vi "Check_and_rewrite_file.vi"(0 "Filename":path, 7 "Present Channels only":bool, 9 "Present Channels":string[](array[string]), 11 "Start of read offset (chars.: 0)":i32) -> (4 "exists?":bool, 6 "Merged Channels":string[](array[string]), 8 "Start of data (bytes)":i32, 10 "No of bytes/row (approx)":i32, 14 "Current file size (bytes)":i32, 15 "Merged?":bool)   [LabVIEW 2014]
uses:
  Anemometry/Anemometry Sub Vis/Globals/Constants_global.vi
panel:
  in  "stop":bool
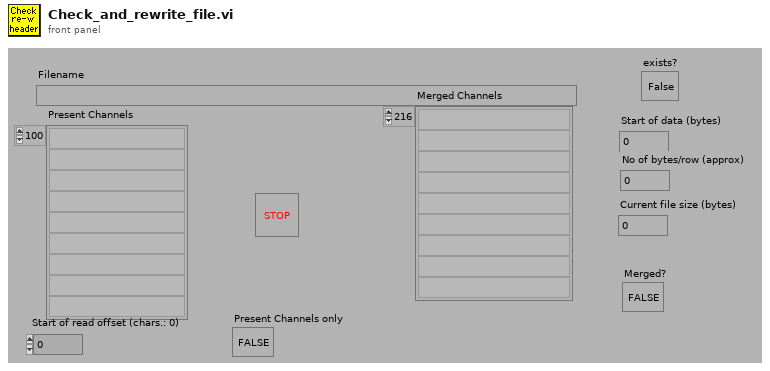
[diagram p1: front panel]
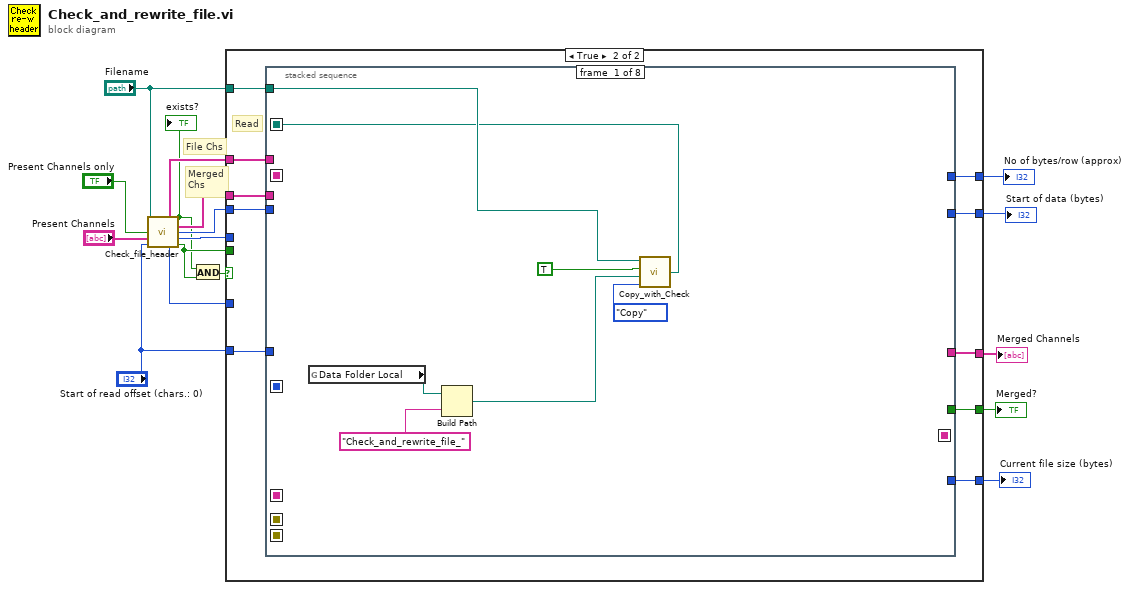
[diagram p0: block diagram]
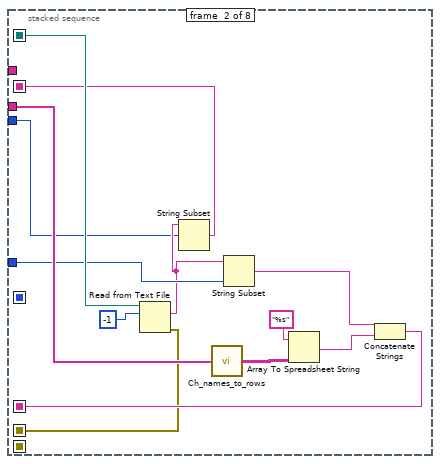
[diagram p3: hidden frame]
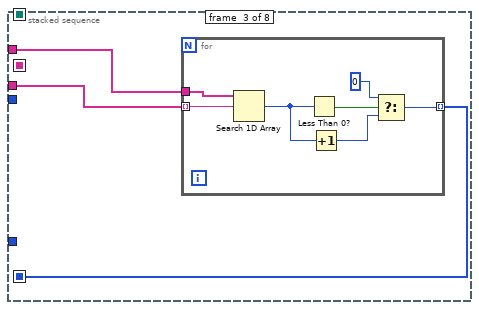
[diagram p4: hidden frame]
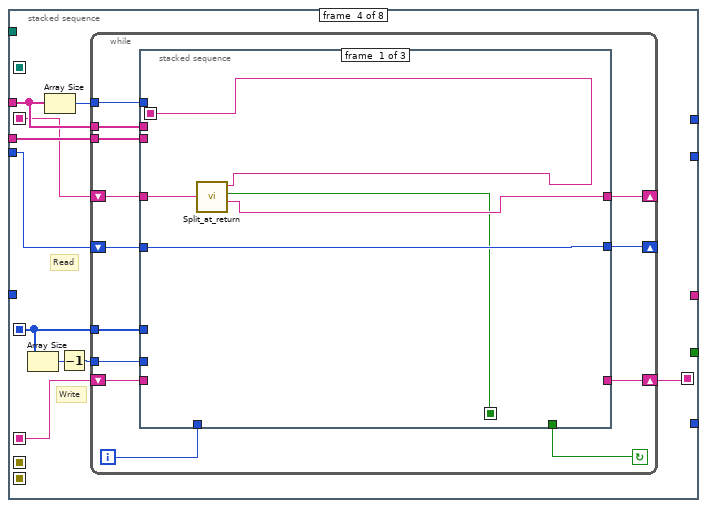
[diagram p5: hidden frame]
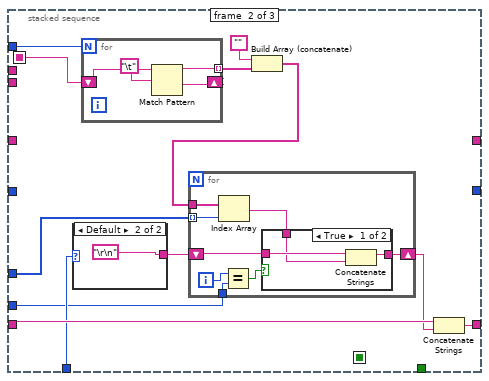
[diagram p6: hidden frame]
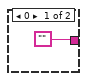
[diagram p7: hidden frame]
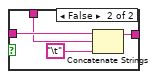
[diagram p8: hidden frame]
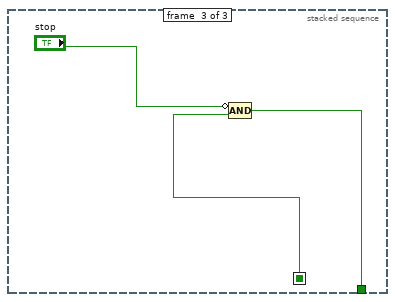
[diagram p9: hidden frame]
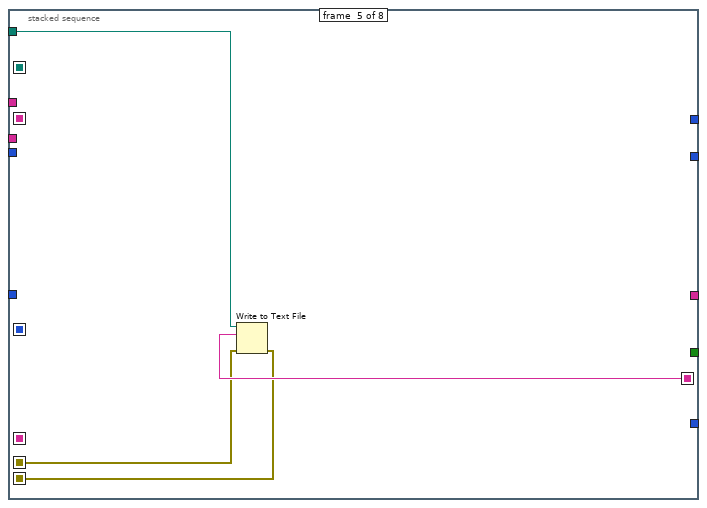
[diagram p10: hidden frame]
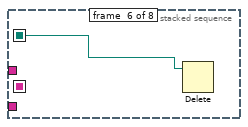
[diagram p11: hidden frame]
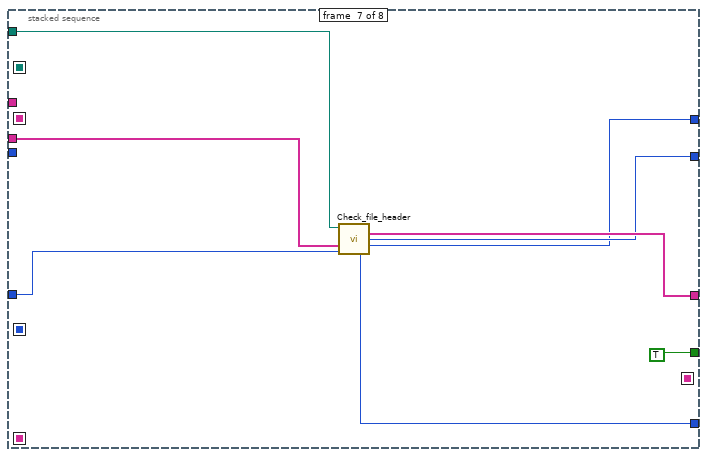
[diagram p12: hidden frame]
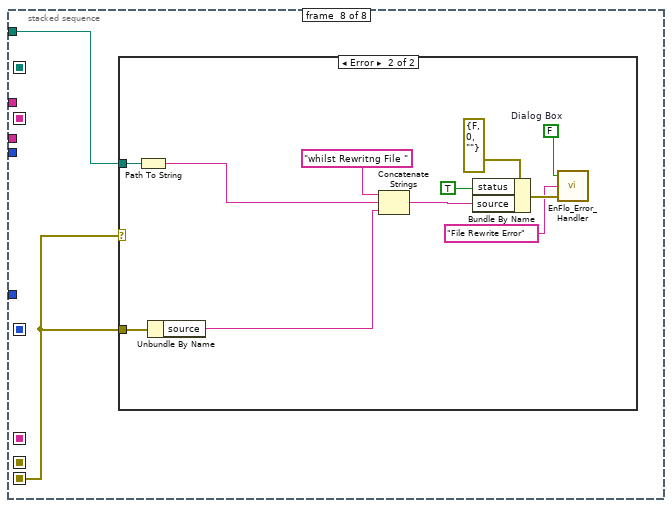
[diagram p13: hidden frame]
diagram:
  # "Merged\nChs"
  # "File Chs"
  n1 = call "Check_file_header.vi"("Filename"="Filename", "Present Channels only"="Present Channels only", "Present Channels"="Present Channels", "Start of read offset (chars.: 0)"="Start of read offset (chars.: 0)") -> ("File Channels"=w5:string[], "exists?"=w4:bool, "Merged Channels"=w11:string[], "Start of data (bytes)"=w10:i32, "No of bytes/row (approx)"=w9:i32, "Current file size (bytes)"=w8:i32, "Merged?"=w12:bool)  [unwired: 5 out]
  "exists?" <- w4
  n2 = And(x=w4, y=w12) -> (x .and. y?=w1:bool)
  n3 = case shown="True" w1 {
    tunnel: [w21 w30] -> w17
    tunnel: [w22 w29] -> w16
    tunnel: [w19 w27] -> w15
    tunnel: [w20 w28] -> w14
    tunnel: [w18 w26] -> w13
    tunnel: w12 -> [w22 _]
    tunnel: w11 -> [w21 w31]
    tunnel: w10 -> [w20 w24]
    tunnel: w9 -> [w19 _]
    tunnel: w8 -> [w18 _]
    tunnel: "Start of read offset (chars.: 0)" -> [_ w25]
    tunnel: w5 -> [_ w23]
    tunnel: "Filename" -> [_ w32]
    frame False {
    }
    frame True {
      # "Read"
      n4 = stacked-sequence {
        seq-local: [w34 _ _ _ _ _ _ _] -> [_ w48 _ _ _ w131 _ _]
        seq-local: [_ _ w53 _ _ _ _ _] -> [_ _ _ w65 _ _ _ _]
        seq-local: [_ _ _ w68 _ _ _ _] -> [_ _ _ _ w130 _ _ _]
        seq-local: [_ w47 _ _ _ _ _ _] -> [_ _ _ w66 _ _ _ _]
        seq-local: [_ w41 _ _ _ _ _ _] -> [_ _ _ w67 _ _ _ _]
        seq-local: [_ w40 _ _ _ _ _ _] -> [_ _ _ _ w128 _ _ _]
        seq-local: [_ _ _ _ w127 _ _ _] -> [_ _ _ _ _ _ _ w140]
        tunnel: w32 -> [w36 _ _ _ w129 _ w138 w141]
        tunnel: w31 -> [_ w50 w55 w69 _ _ w139 _]
        tunnel: [_ _ _ _ _ _ w137 _] -> w30
        tunnel: [_ _ _ _ _ _ TRUE _] -> w29
        tunnel: [_ _ _ _ _ _ w135 _] -> w28
        tunnel: [_ _ _ _ _ _ w134 _] -> w27
        tunnel: [_ _ _ _ _ _ w133 _] -> w26
        tunnel: w25 -> [_ w45 _ _ _ _ w132 _]
        tunnel: w24 -> [_ w42 _ w72 _ _ _ _]
        tunnel: w23 -> [_ _ w54 w70 _ _ _ _]
        frame #0 {
          n5 = global read "Constants_global.vi" "Data Folder Local"() -> (w39:path)
          n6 = Build Path(base path=w39, name or relative path="Check_and_rewrite_file_") -> (appended path=w35:path)
          n7 = call "Copy_with_Check.vi"("Mode"=enum16{"Move", "Copy"}."Copy", "Target Path"=w35, "Variable Target?"=TRUE, "Source Path"=w36) -> ("Pathname Out"=w34:path)
        }
        frame #1 {
          n8 = Read from Text File(file (use dialog)=w48, count=-1) -> (text=w43:string, error out=w40:errorcluster)  [unwired: 2 in, 2 out]
          n9 = String Subset(string=w43, offset (0)=w42) -> (substring=w41:string)  [unwired: 1 in]
          n10 = call "Ch_names_to_rows.vi"("Channel Names"=w50) -> ("3 Row names"=w49:string[][])
          n11 = String Subset(string=w43, length (rest)=w45) -> (substring=w44:string)  [unwired: 1 in]
          n12 = Array To Spreadsheet String(array=w49, 3:"%s" ("format string")) -> (spreadsheet string=w51:string)  [unwired: 1 out]
          n13 = Concatenate Strings(w44, w51) -> (w47:string)
        }
        frame #2 {
          n14 = for {
            tunnel: w54 -> [w62]
            tunnel: w55 -> [w61] mode=indexing
            tunnel: [w56] -> w53 mode=indexing
            n15 = Search 1D Array(1D array=w62, element=w61) -> (index of element=w59:i32)  [unwired: 1 out]
            n16 = Less Than 0?(x=w59) -> (x < 0?=w60:bool)
            n17 = Increment(x=w59) -> (x+1=w58:i32)
            n18 = Select(t=0, s=w60, f=w58) -> (s? t:f=w56:i32)
          }
        }
        frame #3 {
          # "Write"
          # "Read"
          n19 = Array Size(array=w65) -> (size(s)=w64:i32)
          n20 = Array Size(array=w70) -> (size(s)=w71:i32)
          n21 = Decrement(x=w64) -> (x-1=w63:i32)
          n22 = while {
            tunnel: w65 -> [w75]
            tunnel: w69 -> [w79]
            tunnel: w70 -> [w80]
            tunnel: w71 -> [w81]
            shift-left: w66 -> [w78]
            shift-right: [w77] -> w68
            shift-left: w72 -> [w84]
            shift-right: [w83] -> _
            shift-left: w67 -> [w85]
            shift-right: [w82] -> _
            tunnel: w63 -> [w73]
            i -> [w74]
            stop <- w76 continue-if-true
            n23 = stacked-sequence {
              seq-local: [w87 _ _] -> [_ w101 _]
              seq-local: [w86 _ _] -> [_ _ w124]
              tunnel: w85 -> [w89 _ _]
              tunnel: w84 -> [w90 _ _]
              tunnel: [w90 _ _] -> w83
              tunnel: [w88 _ _] -> w82
              tunnel: w81 -> [_ w102 _]
              tunnel: w80 -> [_ _ _]
              tunnel: w79 -> [_ _ _]
              tunnel: w78 -> [_ w94 _]
              tunnel: [_ w95 _] -> w77
              tunnel: [_ _ w125] -> w76
              tunnel: w75 -> [_ w97 _]
              tunnel: w74 -> [_ w92 _]
              tunnel: w73 -> [_ w91 _]
              frame #0 {
                n24 = call "Split_at_return.vi"("String"=w89) -> ("before substring"=w87:string, "Matched?"=w86:bool, "after substring"=w88:string)  [unwired: 1 in, 1 out]
              }
              frame #1 {
                n25 = case shown="Default" w92 {
                  tunnel: ["" "\r\n"] -> w96
                  frame 0 {
                  }
                  frame Default {
                  }
                }
                n26 = for {
                  N: w102 -> [_]
                  shift-right: [w121] -> _
                  shift-left: w101 -> [w122]
                  tunnel: [w120] -> w99 mode=indexing
                  n27 = Match Pattern(string=w122, regular expression="\t") -> (before substring=w120:string, after substring=w121:string)  [unwired: 3 out]
                }
                n28 = Build Array (concatenate)("", w99) -> (w98:string[])
                n29 = for {
                  tunnel: w97 -> [w112] mode=indexing
                  tunnel: w98 -> [w111]
                  shift-right: [w108] -> w93
                  shift-left: w96 -> [w110]
                  tunnel: w91 -> [w107]
                  i -> [w106]
                  n30 = Index Array(array=w111, index=w112) -> (element=w109:string)
                  n31 = Equal?(x=w106, y=w107) -> (x = y?=w105:bool)
                  n32 = case shown="True" w105 {
                    tunnel: w110 -> [w115 w119]
                    tunnel: w109 -> [w114 w118]
                    tunnel: [w113 w117] -> w108
                    frame True {
                      n33 = Concatenate Strings(w115, w114) -> (w113:string)
                    }
                    frame False {
                      n34 = Concatenate Strings(w119, w118, "\t") -> (w117:string)
                    }
                  }
                }
                n35 = Concatenate Strings(w94, w93) -> (w95:string)
              }
              frame #2 {
                n36 = Compound Arithmetic op=AND(invert "stop", w124) -> (w125:bool)
              }
            }
          }
        }
        frame #4 {
          n37 = Write to Text File(file (use dialog)=w129, text=w130, error in=w128) -> (error out=w127:errorcluster)  [unwired: 1 in, 2 out]
        }
        frame #5 {
          n38 = Delete(path (use dialog)=w131) -> ()  [unwired: 1 in, 6 out]
        }
        frame #6 {
          n39 = call "Check_file_header.vi"("Filename"=w138, "Present Channels"=w139, "Start of read offset (chars.: 0)"=w132) -> ("Merged Channels"=w137:string[], "Start of data (bytes)"=w135:i32, "No of bytes/row (approx)"=w134:i32, "Current file size (bytes)"=w133:i32)  [unwired: 1 in, 8 out]
        }
        frame #7 {
          n40 = case shown="Error" w140 {
            tunnel: w141 -> [_ w146]
            tunnel: w140 -> [_ w143]
            frame No Error {
            }
            frame Error {
              w149 = FALSE  # Dialog Box
              n41 = Path To String(path=w146) -> (string=w145:string)
              n42 = Unbundle By Name(w143) -> ("source"=w142:string)
              n43 = Concatenate Strings("whilst Rewritng File ", w145, w142) -> (w147:string)
              n44 = Bundle By Name(cluster=errorcluster {"status"=FALSE, "code"=0, "source"=""} ("error in (no error)"), "status"=TRUE ("Bundle Element"), "source"=w147) -> (w150:errorcluster)
              n45 = call "EnFlo_Error_Handler.vi"("error in (no error)"=w150, "Error Type"="File Rewrite Error", "Dialog Box (T)"=w149) -> ()  [unwired: 3 out]
            }
          }
        }
      }
    }
  }
  "Merged?" <- w16
  "Merged Channels" <- w17
  "Current file size (bytes)" <- w13
  "Start of data (bytes)" <- w14
  "No of bytes/row (approx)" <- w15
